vi "Set Re-entrancy for VIs in a Folder.vi"(8 "error in (no error)":errorcluster, 9 "Reentrancy Type":T1(ring), 10 "Is Reentrant?":bool, 11 "VI Folder":path) -> (0 "error out":errorcluster, 3 "VI List":path[](array[path]))   [LabVIEW 2014, in "SLL Application.lvlib"]
doc: "This VI can be used to find the list of broken VIs in a folder. This also returns VIs which are of higher LabVIEW version than the currently used LabVIEW version."
uses:
  SLL Application.lvlib
panel:
  out "VIs with Errors":path[](array[path])
  out "Progress":i32
  # "Note: Polymorphic VIs will result in error when setting the re-entrancy setting."
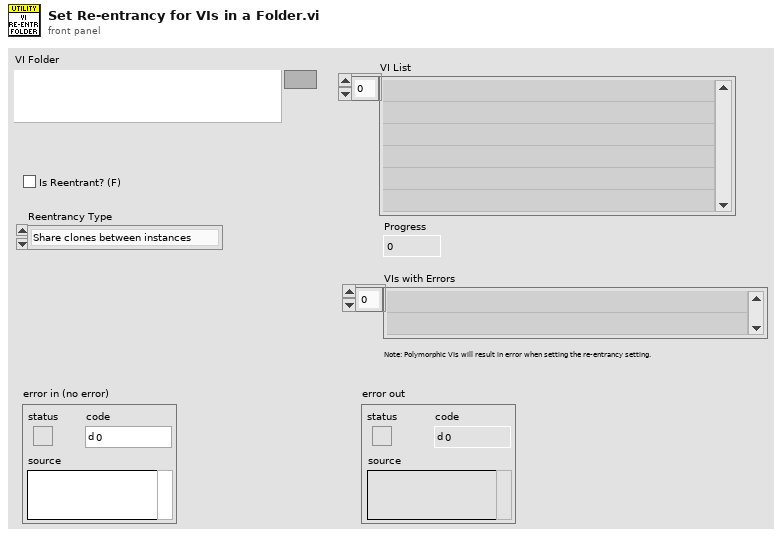
[diagram p1: front panel]
types:
  T1 = enum16{"Share clones between instances", "Preallocate clone for each instance"}
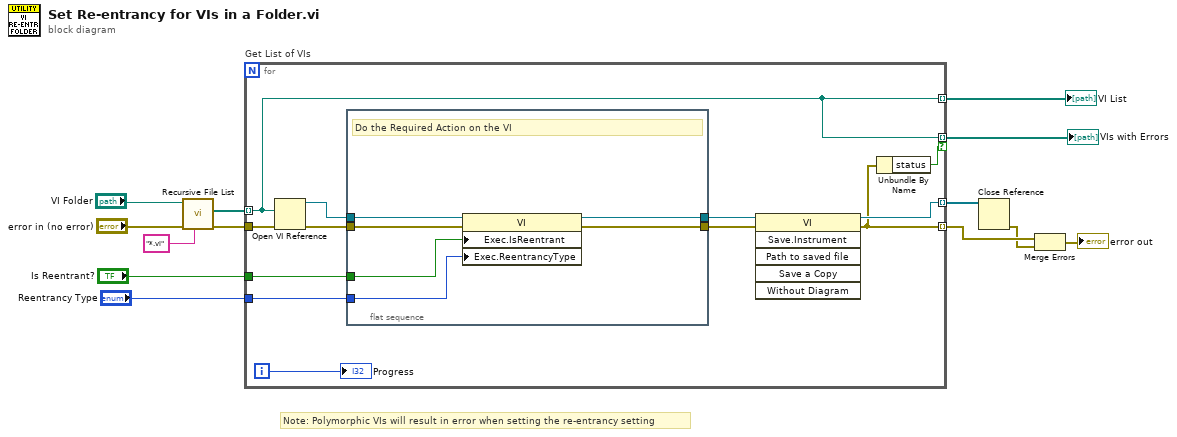
[diagram p0: block diagram]
diagram:
  # "Note: Polymorphic VIs will result in error when setting the re-entrancy setting"
  n1 = call <vilib>:"Recursive File List.vi"("pattern"="*.vi", "error in (no error)"="error in (no error)", "Folder Path"="VI Folder") -> ("error out"=w7:errorcluster, "All Files in Dir"=w10:path[])  [unwired: 4 in, 3 out]
  n2 = for "Get List of VIs" {
    tunnel: [w19] -> w13 mode=indexing
    tunnel: w10 -> [w16] mode=indexing
    tunnel: [w16] -> w9 mode=indexing
    tunnel: w7 -> [w24]
    tunnel: [w15] -> w6 mode=indexing
    tunnel: "Reentrancy Type" -> [w18]
    tunnel: "Is Reentrant?" -> [w17]
    tunnel: [w16] -> w1 mode=indexing if=w14
    i -> [w21]
    n3 = Open VI Reference(vi path=w16, error in (no error)=w24) -> (vi reference=w25:refnum<vi>, error out=w23:errorcluster)  [unwired: 4 in]
    n4 = flat-sequence {
      tunnel: w25 -> [w26]
      tunnel: w23 -> [w31]
      tunnel: [w30] -> w22
      tunnel: [w29] -> w20
      tunnel: w18 -> [w28]
      tunnel: w17 -> [w27]
      frame #0 {
        # "Do the Required Action on the VI"
        n5 = property class="VI"(reference=w26, error in=w31, "Exec.IsReentrant"=w27, "Exec.ReentrancyType"=w28) -> (reference out=w29:refnum<vi>, error out=w30:errorcluster)
      }
    }
    n6 = invoke class="VI" method="Save.Instrument"(reference=w20, error in=w22) -> (reference out=w19:refnum<vi>, error out=w15:errorcluster)  [unwired: 4 in, 4 out]
    n7 = Unbundle By Name(w15) -> ("status"=w14:bool)
    "Progress" <- w21
  }
  "VI List" <- w9
  "VIs with Errors" <- w1
  n8 = Close Reference(reference=w13) -> (error out=w5:errorcluster)  [unwired: 1 in]
  n9 = Merge Errors(w6, w5) -> (→"error out":errorcluster)
